vi "4. FGV Cmd check.vi"(8 "error in (no error)":errorcluster, 11 "VISA resource name":refnum<visa-resource-name>="COM3") -> (0 "error out":errorcluster, 1 "Checksum":u32, 2 "Command type (ACK, NACK, Normal)":i32, 3 "Command":string)   [LabVIEW 2014]
uses:
  control/FGV Serial Tasks.ctl
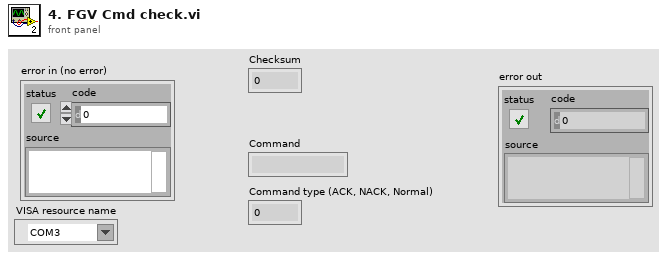
[diagram p1: front panel]
types:
  T1 = typedef "FGV Serial Tasks.ctl" = enum16{"Open", "Read", "Write", "Close", "Flush"}
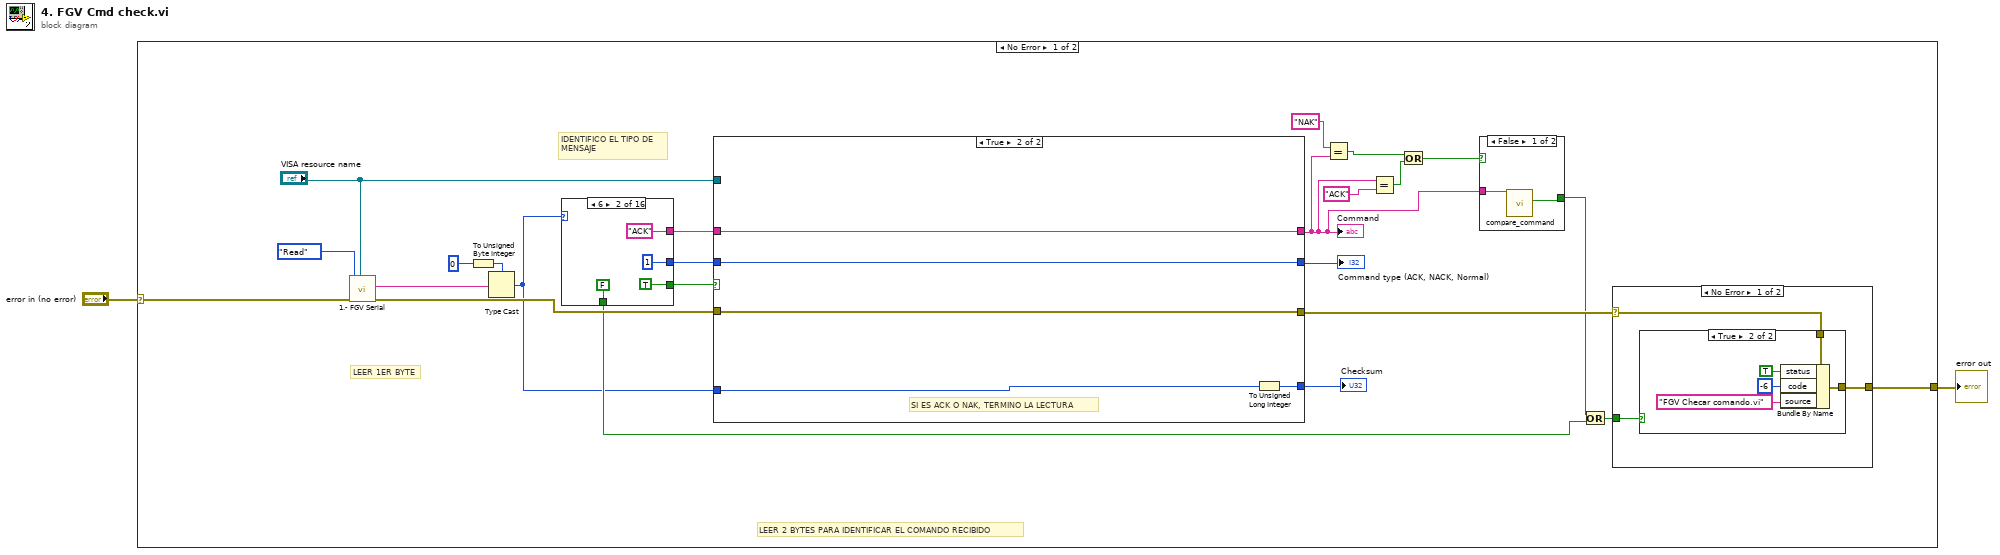
[diagram p0: block diagram]
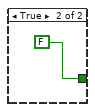
[diagram p2: hidden frame]
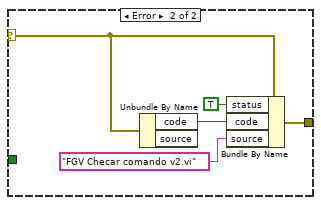
[diagram p4: hidden frame]
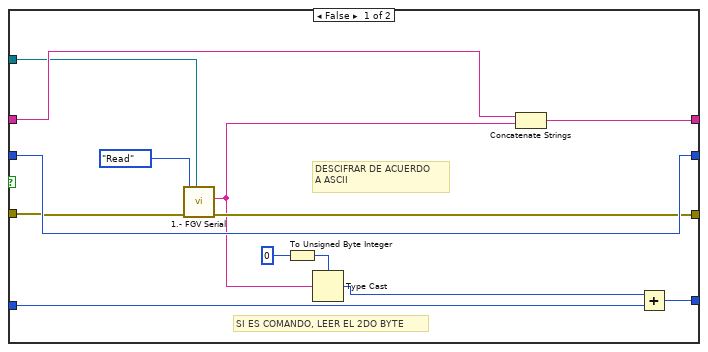
[diagram p5: hidden frame]
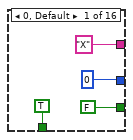
[diagram p6: hidden frame]
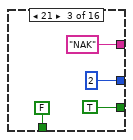
[diagram p7: hidden frame]
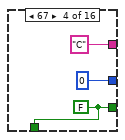
[diagram p8: hidden frame]
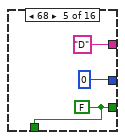
[diagram p9: hidden frame]
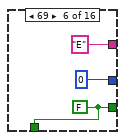
[diagram p10: hidden frame]
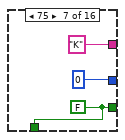
[diagram p11: hidden frame]
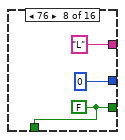
[diagram p12: hidden frame]
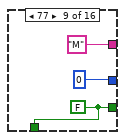
[diagram p13: hidden frame]
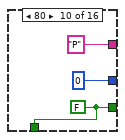
[diagram p14: hidden frame]
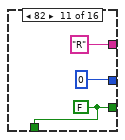
[diagram p15: hidden frame]
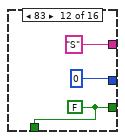
[diagram p16: hidden frame]
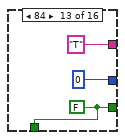
[diagram p17: hidden frame]
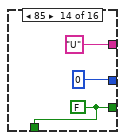
[diagram p18: hidden frame]
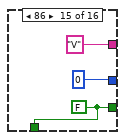
[diagram p19: hidden frame]
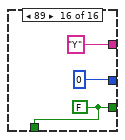
[diagram p20: hidden frame]
diagram:
  n1 = case shown="No Error" "error in (no error)" {
    selector: "error in (no error)" -> [w26 w113]
    tunnel: [w21 w113] -> w1
    frame No Error {
      # "IDENTIFICO EL TIPO DE\nMENSAJE"
      # "LEER 1ER BYTE"
      # "LEER 2 BYTES PARA IDENTIFICAR EL COMANDO RECIBIDO"
      n2 = call "1.- FGV Serial.vi"("VISA resource name"="VISA resource name", "error in (no error)"=w26, "Task"=FGV_Serial_Tasks."Read") -> ("error out"=w22:errorcluster, "Receive buffer"=w3:string)  [unwired: 6 in, 1 out]
      n3 = To Unsigned Byte Integer(number=u8 0) -> (unsigned 8bit integer=w16:u8)
      n4 = Type Cast(type=w16, x=w3) -> (*(type *) &x=w19:u8)
      n5 = case shown="6" w19 {
        tunnel: ["X" "ACK" "NAK" "C" "D" "E" "K" "L" "M" "P" "R" "S" "T" "U" "V" "Y"] -> w25
        tunnel: [0 ("Status") 1 ("Status") 2 ("Status") 0 ("Status") 0 ("Status") 0 ("Status") 0 ("Status") 0 ("Status") 0 ("Status") 0 ("Status") 0 ("Status") 0 ("Status") 0 ("Status") 0 ("Status") 0 ("Status") 0 ("Status")] -> w24
        tunnel: [FALSE TRUE TRUE w74 w77 w80 w83 w86 w89 w92 w95 w98 w101 w104 w107 w110] -> w23
        tunnel: [TRUE FALSE FALSE w74 w77 w80 w83 w86 w89 w92 w95 w98 w101 w104 w107 w110] -> w20
        frame 0, Default {
        }
        frame 6 {
        }
        frame 21 {
        }
        frame 67 {
          w74 = FALSE
        }
        frame 68 {
          w77 = FALSE
        }
        frame 69 {
          w80 = FALSE
        }
        frame 75 {
          w83 = FALSE
        }
        frame 76 {
          w86 = FALSE
        }
        frame 77 {
          w89 = FALSE
        }
        frame 80 {
          w92 = FALSE
        }
        frame 82 {
          w95 = FALSE
        }
        frame 83 {
          w98 = FALSE
        }
        frame 84 {
          w101 = FALSE
        }
        frame 85 {
          w104 = FALSE
        }
        frame 86 {
          w107 = FALSE
        }
        frame 89 {
          w110 = FALSE
        }
      }
      n6 = case shown="True" w23 {
        tunnel: [w56 w61] -> w4
        tunnel: w25 -> [w55 w61]
        tunnel: [w54 w60] -> w14
        tunnel: w24 -> [w54 w60]
        tunnel: w22 -> [w53 w59]
        tunnel: [w52 w59] -> w12
        tunnel: [w51 w58] -> w13
        tunnel: w19 -> [w46 w57]
        tunnel: "VISA resource name" -> [w44 _]
        frame False {
          # "DESCIFRAR DE ACUERDO\nA ASCII"
          # "SI ES COMANDO, LEER EL 2DO BYTE"
          n7 = call "1.- FGV Serial.vi"("VISA resource name"=w44, "error in (no error)"=w53, "Task"=FGV_Serial_Tasks."Read") -> ("error out"=w52:errorcluster, "Receive buffer"=w48:string)  [unwired: 6 in, 1 out]
          n8 = To Unsigned Byte Integer(number=u8 0) -> (unsigned 8bit integer=w49:u8)
          n9 = Type Cast(type=w49, x=w48) -> (*(type *) &x=w47:u8)
          n10 = Concatenate Strings(w55, w48) -> (w56:string)
          n11 = Add(x=w47, y=w46) -> (x+y=w51:u8)
        }
        frame True {
          # "SI ES ACK O NAK, TERMINO LA LECTURA"
          n12 = To Unsigned Long Integer(number=w57) -> (unsigned 32bit integer=w58:u32)
        }
      }
      "Command" <- w4
      "Command type (ACK, NACK, Normal)" <- w14
      "Checksum" <- w13
      n13 = Equal?(x="NAK", y=w4) -> (x = y?=w6:bool)
      n14 = Equal?(x=w4, y="ACK") -> (x = y?=w5:bool)
      n15 = Or(x=w6, y=w5) -> (x .or. y?=w7:bool)
      n16 = case shown="False" w7 {
        tunnel: [w28 FALSE ("Comando no reconocido")] -> w10
        tunnel: w4 -> [w27 _]
        frame False {
          n17 = call "compare_command.vi"("Command"=w27) -> ("Unknown"=w28:bool)  [unwired: 9 in, 1 out]
        }
        frame True {
        }
      }
      n18 = Or(x=w10, y=w20) -> (x .or. y?=w11:bool)
      n19 = case shown="No Error" w12 {
        selector: w12 -> [w32 w42]
        tunnel: [w31 w41] -> w21
        tunnel: w11 -> [w30 _]
        frame No Error {
          n20 = case shown="True" w30 {
            tunnel: w32 -> [w33 w38]
            tunnel: [w33 w37] -> w31
            frame False {
            }
            frame True {
              n21 = Bundle By Name(cluster=w38, "status"=TRUE, "code"=-6, "source"="FGV Checar comando.vi") -> (w37:errorcluster)
            }
          }
        }
        frame Error {
          n22 = Unbundle By Name(w42) -> ("code"=w43:i32)  [unwired: 1 out]
          n23 = Bundle By Name(cluster=w42, "status"=TRUE, "code"=w43, "source"="FGV Checar comando v2.vi") -> (w41:errorcluster)
        }
      }
    }
    frame Error {
    }
  }
  "error out" <- w1
